vi "ReadUserLog.vi"(5 "Username":string, 7 "file path (use dialog)":path) -> (0 "Level":dbl, 1 "Score":dbl, 2 "Hashed Password":string, 3 "Found?":bool)   [LabVIEW 2025]
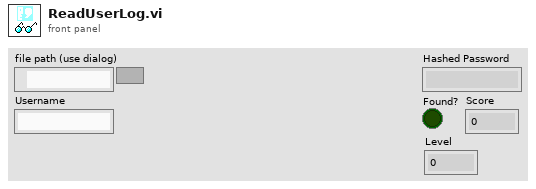
[diagram p1: front panel]
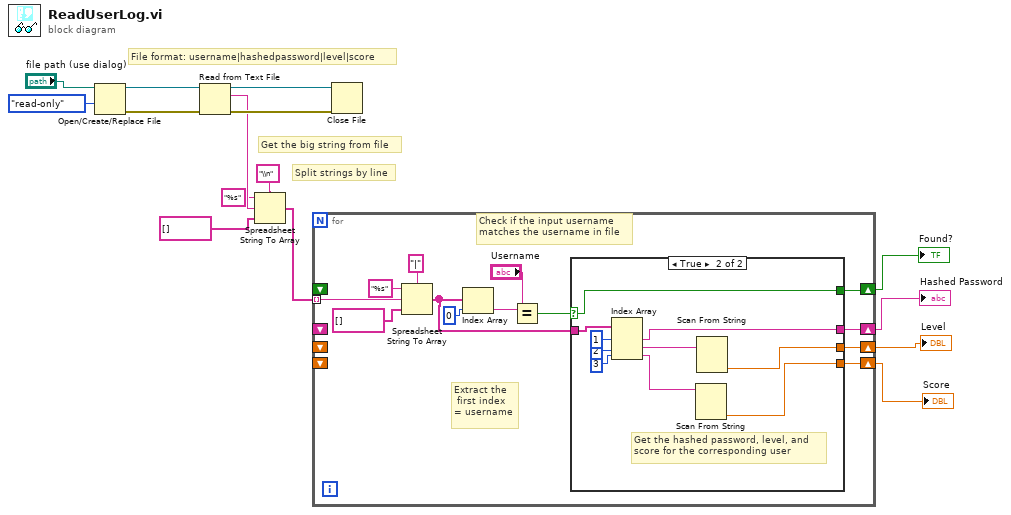
[diagram p0: block diagram]
diagram:
  # "File format: username|hashedpassword|level|score"
  # "Split strings by line"
  # "Get the big string from file"
  n1 = Open/Create/Replace File(file path (use dialog)="file path (use dialog)", access (0:read/write)=enum16{"read/write", "read-only", "write-only"}."read-only") -> (refnum out=w13:refnum<file>, error out=w14:errorcluster)  [unwired: 4 in, 1 out]
  n2 = Read from Text File(file (use dialog)=w13, error in=w14) -> (refnum out=w11:refnum<file>, text=w10:string, error out=w12:errorcluster)  [unwired: 2 in, 1 out]
  n3 = Spreadsheet String To Array(delimiter (Tab)="\\n", format string="%s", spreadsheet string=w10, array type (2D Dbl)=string[] []) -> (array=w7:string[])
  n4 = for {
    tunnel: w7 -> [w28] mode=indexing
    shift-right: [w21] -> w6
    shift-left: _ -> [_]
    shift-right: [w20] -> w3
    shift-left: _ -> [_]
    shift-right: [w19] -> w4
    shift-left: _ -> [_]
    shift-right: [w17] -> w5
    shift-left: _ -> [_]
    # "Check if the input username\nmatches the username in file"
    # "Extract the\n first index \n= username"
    n5 = Spreadsheet String To Array(delimiter (Tab)="|", format string="%s", spreadsheet string=w28, array type (2D Dbl)=string[] []) -> (array=w22:string[])
    n6 = Index Array(array=w22, index=0) -> (element=w24:string)
    n7 = Equal?(x=w24, y="Username") -> (x = y?=w18:bool)
    n8 = case shown="True" w18 {
      selector: w18 -> [_ w33]
      tunnel: w22 -> [_ w38]
      tunnel: [_ w34] -> w21
      tunnel: [_ w31] -> w20
      tunnel: [_ w29] -> w19
      tunnel: [_ w33] -> w17
      frame False {
      }
      frame True {
        # "Get the hashed password, level, and \nscore for the corresponding user"
        n9 = Index Array(array=w38, index #1=1 ("index"), index #2=2 ("index"), index #3=3 ("index")) -> (element #1=w34:string, element #2=w32:string, element #3=w30:string)
        n10 = Scan From String(input string=w30) -> (output 1=w29:dbl)  [unwired: 4 in, 3 out]
        n11 = Scan From String(input string=w32) -> (output 1=w31:dbl)  [unwired: 4 in, 3 out]
      }
    }
  }
  "Hashed Password" <- w6
  "Found?" <- w5
  "Score" <- w4
  "Level" <- w3
  n12 = Close File(refnum=w11, error in=w12) -> ()  [unwired: 2 out]
